vi "解压缩.vi"(8 "error in (no error)":errorcluster caption="错误输入（无错误）", 11 "Zip file":path caption="Zip文件") -> (0 "error out":errorcluster, 2 "MD5":string, 3 "待校验的文件路径":path)   [LabVIEW 2016, in "数据传输系统-03.lvlib" / "update.lvlib"]
uses:
  update.lvlib
  <vilib>/zip/NI_Unzip.lvlib
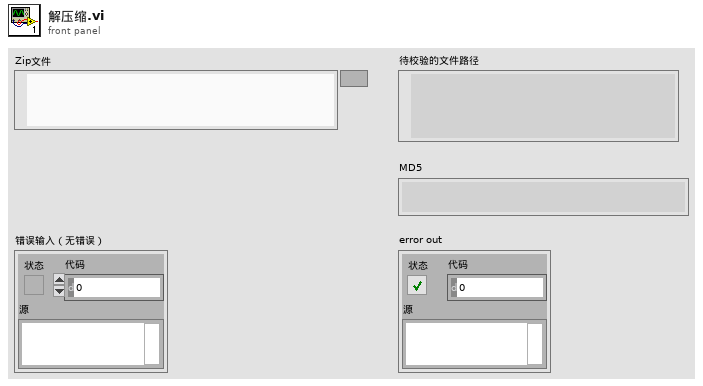
[diagram p1: front panel]
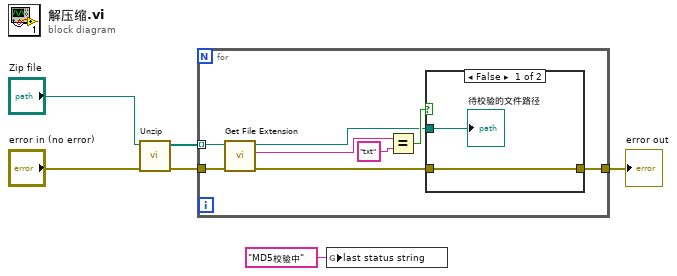
[diagram p0: block diagram]
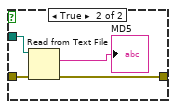
[diagram p2: hidden frame]
diagram:
  n1 = call <vilib>:"Unzip.vi"("error in (no error)"="error in (no error)", "Zip file"="Zip file") -> ("error out"=w4:errorcluster, "Unzipped files"=w5:path[])  [unwired: 7 in, 1 out]
  n2 = for {
    tunnel: w5 -> [w14] mode=indexing
    tunnel: w4 -> [w13]
    tunnel: [w7] -> w3
    n3 = call <vilib>:"Get File Extension.vi"("error in (no error)"=w13, "file"=w14) -> ("error out"=w8:errorcluster, "lowercase file extension"=w12:string, "dup file"=w9:path)  [unwired: 5 in, 2 out]
    n4 = Equal?(x=w12, y="txt") -> (x = y?=w10:bool)
    n5 = case shown="False" w10 {
      tunnel: w9 -> [w16 w20]
      tunnel: w8 -> [w15 w19]
      tunnel: [w15 w17] -> w7
      frame False {
        "待校验的文件路径" <- w16
      }
      frame True {
        n6 = Read from Text File(file (use dialog)=w20, error in=w19) -> (text=→"MD5":string, error out=w17:errorcluster)  [unwired: 2 in, 2 out]
      }
    }
  }
  "error out" <- w3
  n7 = global write "更新全局变量.vi" "last status string"("MD5校验中" ("last status string")) -> ()
